vi "Obtain Enum Queue.vi"(8 "error in":errorcluster, 11 "Name":string) -> (0 "error out":errorcluster, 3 "Queue Out":refnum<queue>)   [LabVIEW 2020, in "Enum Queue State Machine.lvlib"]
uses:
  Enum Queue State Machine.lvlib
  Controls/Enum Message.ctl
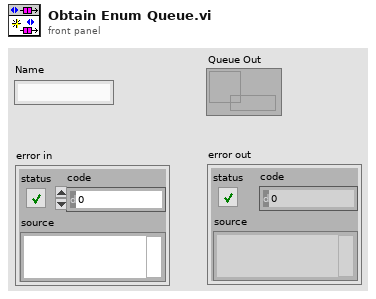
[diagram p1: front panel]
types:
  T1 = typedef "Enum Queue State Machine.lvlib/Enum Message.ctl" = cluster{"State":i32, "Data":variant}
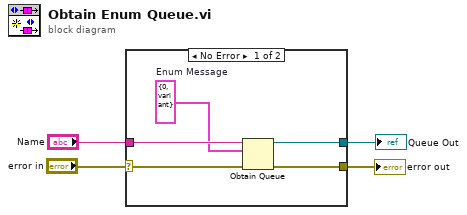
[diagram p0: block diagram]
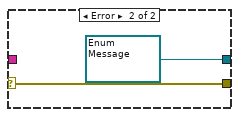
[diagram p2: hidden frame]
diagram:
  n1 = case shown="No Error" "error in" {
    selector: "error in" -> [w9 w11]
    tunnel: [w8 w11] -> w3
    tunnel: "Name" -> [w7 _]
    tunnel: [w6 refnum<queue> refnum ("queue out")] -> w1
    frame No Error {
      w5 = T1 {"State"=0, "Data"=variant}  # Enum Message
      n2 = Obtain Queue(name (unnamed)=w7, element data type=w5, error in (no error)=w9) -> (queue out=w6:refnum<queue>, error out=w8:errorcluster)  [unwired: 2 in, 1 out]
    }
    frame Error {
    }
  }
  "error out" <- w3
  "Queue Out" <- w1
